vi "TrapsMachMitteln.vi"(1 "Traps/MachKoeff0":dbl[](array[numeric]), 2 "Traps/MachKoeff1":dbl[](array[numeric]), 3 "Traps/MachKoeff2":dbl[](array[numeric]), 4 "FPGA VI Reference In":refnum<k20>) -> ()   [LabVIEW 2010]
uses:
  <vilib>/rvi/interface/nirviReadWriteControl/nirviReadWriteControl.xnode
  C:/Users/HAGAR-IV/Desktop/Zeugs/markus/version feb 2012/FPGA Bitfiles/pertrasgcfpga2_FPGATarget_FPGA-Programm-10_16368CB6.lvbitx
  C:/Users/HAGAR-IV/Desktop/Zeugs/Johnny/pertrasgc fpga/FPGA-Programm-10-14.vi
  <vilib>/rvi/interface/common/niFpgaNodeNameForErrorReporting.ctl
  <vilib>/rvi/errors/niLvFpgaWhatHappensToTopLevelVI.ctl
  GVTrapsMachs.vi
  <vilib>/Utility/error.llb/Error Cluster From Error Code.vi
  <vilib>/rvi/errors/niLvFpgaAdjustHostInterfaceError.vi
  NiFpgaLv.dll
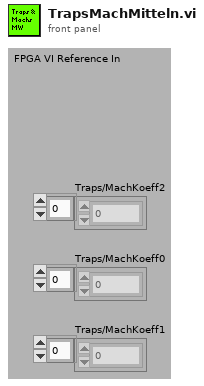
[diagram p1: front panel]
types:
  T1 = typedef "niFpgaNodeNameForErrorReporting.ctl" = enum16{"Open FPGA VI Reference", "Read/Write Control", "Invoke Method: Abort", "Invoke Method: Acknowledge IRQ", "Invoke Method: Download", "Invoke Method: FIFO.Configure", "Invoke Method: FIFO.Read", "Invoke Method: FIFO.Start", "Invoke Method: FIFO.Stop", "Invoke Method: FIFO.Write", "Invoke Method: Reset", "Invoke Method: Run", "Invoke Method: Wait on IRQ", "Close FPGA VI Reference"}
  T2 = typedef "niLvFpgaWhatHappensToTopLevelVI.ctl" = enum16{"top level VI scripted behind XNode", "top level VI inlined behind XNode"}
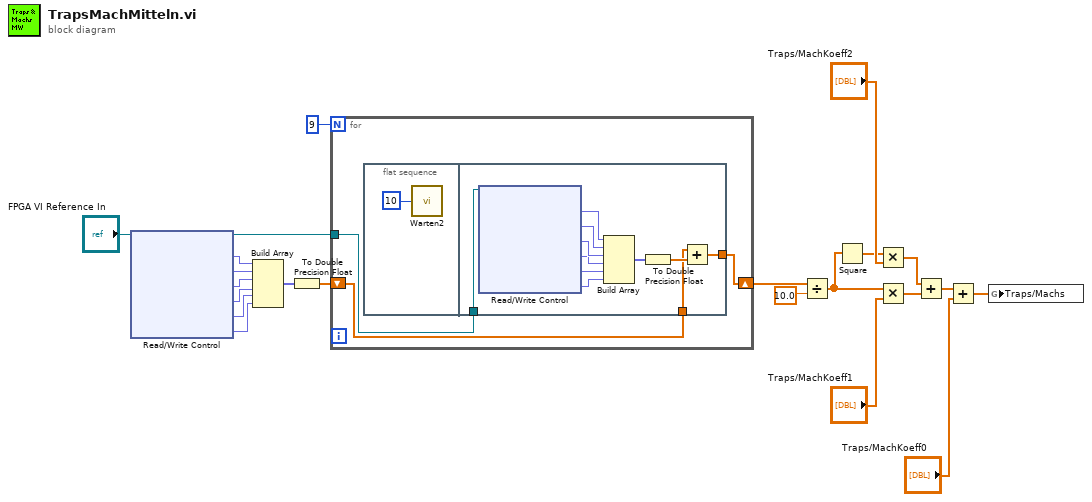
[diagram p0: block diagram]
diagram:
  n1 = xnode "Read/Write Control"("FPGA VI Reference In"="FPGA VI Reference In") -> ("FPGA VI Reference Out"=w12:refnum<k20>, "UWidr[V]Trap1"=w13:fxp<+/-,16,4>, "UTemp[V]Trap1"=w14:fxp<+/-,16,4>, "UWidr[V]Trap2"=w15:fxp<+/-,16,4>, "UTemp[V]Trap2"=w16:fxp<+/-,16,4>, "U[V]Mach1"=w17:fxp<+/-,16,4>, "U[V]Mach2"=w18:fxp<+/-,16,4>)  [unwired: 1 in, 1 out]
  n2 = Build Array(w13, w14, w15, w16, w17, w18) -> (w3:fxp<+/-,16,4>[])
  n3 = To Double Precision Float(number=w3) -> (double precision float=w19:dbl[])
  n4 = for {
    N: 9 -> [_]
    tunnel: w12 -> [w25]
    shift-right: [w23] -> w10
    shift-left: w19 -> [w24]
    n5 = flat-sequence {
      tunnel: w25 -> [w37]
      tunnel: w24 -> [w28]
      tunnel: [w27] -> w23
      frame #0 {
        n6 = call "Warten2"("Count(mSec)"=u32 10) -> ()  [unwired: 1 out]
      }
      frame #1 {
        n7 = xnode "Read/Write Control"("FPGA VI Reference In"=w37) -> ("UWidr[V]Trap1"=w36:fxp<+/-,16,4>, "UTemp[V]Trap1"=w35:fxp<+/-,16,4>, "UWidr[V]Trap2"=w34:fxp<+/-,16,4>, "UTemp[V]Trap2"=w33:fxp<+/-,16,4>, "U[V]Mach1"=w32:fxp<+/-,16,4>, "U[V]Mach2"=w31:fxp<+/-,16,4>)  [unwired: 1 in, 2 out]
        n8 = Build Array(w36, w35, w34, w33, w32, w31) -> (w30:fxp<+/-,16,4>[])
        n9 = To Double Precision Float(number=w30) -> (double precision float=w29:dbl[])
        n10 = Add(x=w28, y=w29) -> (x+y=w27:dbl[])
      }
    }
  }
  n11 = Divide(x=w10, y=10.0) -> (x/y=w5:dbl[])
  n12 = Square(x=w5) -> (x^2=w6:dbl[])
  n13 = Multiply(x=w6, y="Traps/MachKoeff2") -> (x*y=w7:dbl[])
  n14 = Multiply(x=w5, y="Traps/MachKoeff1") -> (x*y=w8:dbl[])
  n15 = Add(x=w7, y=w8) -> (x+y=w9:dbl[])
  n16 = Add(x=w9, y="Traps/MachKoeff0") -> (x+y=w1:dbl[])
  n17 = global write "GVTrapsMachs.vi" "Traps/Machs"(w1) -> ()
